vi "Parse Project Based Analysis.vi"(8 "error in (no error)":errorcluster, 11 "Element in":refnum<k20>) -> (0 "error out":errorcluster, 2 "Project Based Analysis":T1, 3 "Element out":refnum<k20>)   [LabVIEW 2020]
uses:
  <vilib>/xml/Close Reference(Node).vi
  <vilib>/xml/NI_XML.lvlib
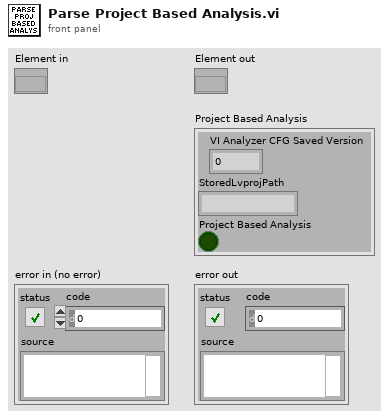
[diagram p1: front panel]
types:
  T1 = cluster{"VI Analyzer CFG Saved Version":u16, "StoredLvprojPath":string, "Project Based Analysis":bool}
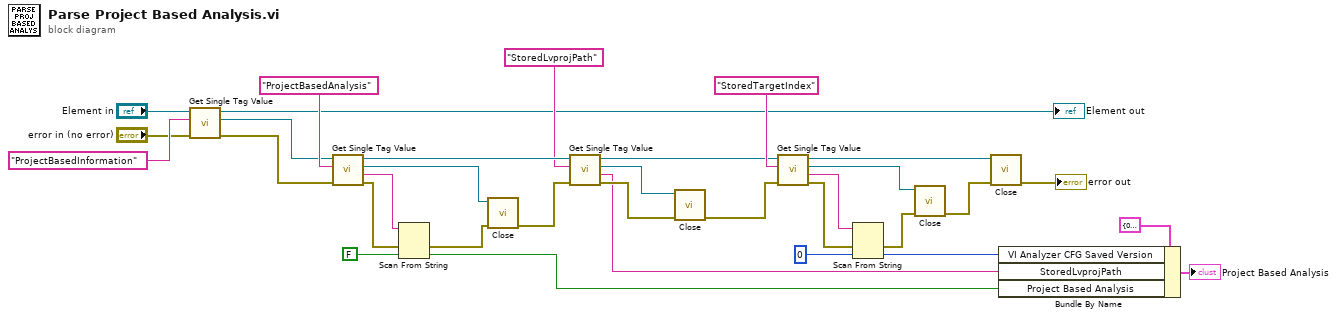
[diagram p0: block diagram]
diagram:
  n1 = call <vilib>:"Get Single Tag Value.vi"("Error In"="error in (no error)", "Tag Name"="ProjectBasedInformation", "Element In"="Element in") -> ("Error Out"=w2:errorcluster, "Tag Reference"=w5:refnum<k20>, "Element Out"=→"Element out":refnum<k20>)  [unwired: 5 in, 1 out]
  n2 = call <vilib>:"Get Single Tag Value.vi"("Error In"=w2, "Tag Name"="ProjectBasedAnalysis", "Element In"=w5) -> ("Error Out"=w18:errorcluster, "Tag Value"=w23:string, "Tag Reference"=w33:refnum<k20>, "Element Out"=w15:refnum<k20>)  [unwired: 5 in]
  n3 = Scan From String(input string=w23, error in=w18, default 1=FALSE) -> (error out=w31:errorcluster, output 1=w9:bool)  [unwired: 2 in, 2 out]
  n4 = call-poly <vilib>:"Close.vi"("error in (no error)"=w31, "node"=w33) -> ("error out"=w32:errorcluster)  [unwired: 7 in]
  n5 = call <vilib>:"Get Single Tag Value.vi"("Error In"=w32, "Tag Name"="StoredLvprojPath", "Element In"=w15) -> ("Error Out"=w26:errorcluster, "Tag Value"=w10:string, "Tag Reference"=w25:refnum<k20>, "Element Out"=w16:refnum<k20>)  [unwired: 5 in]
  n6 = call-poly <vilib>:"Close.vi"("error in (no error)"=w26, "node"=w25) -> ("error out"=w30:errorcluster)  [unwired: 7 in]
  n7 = call <vilib>:"Get Single Tag Value.vi"("Error In"=w30, "Tag Name"="StoredTargetIndex", "Element In"=w16) -> ("Error Out"=w20:errorcluster, "Tag Value"=w24:string, "Tag Reference"=w29:refnum<k20>, "Element Out"=w22:refnum<k20>)  [unwired: 5 in]
  n8 = Scan From String(input string=w24, error in=w20, default 1=u16 0 ("VI Analyzer CFG Saved Version")) -> (error out=w27:errorcluster, output 1=w11:u16)  [unwired: 2 in, 2 out]
  n9 = call-poly <vilib>:"Close.vi"("error in (no error)"=w27, "node"=w29) -> ("error out"=w28:errorcluster)  [unwired: 7 in]
  n10 = call-poly <vilib>:"Close.vi"("error in (no error)"=w28, "node"=w22) -> ("error out"=→"error out":errorcluster)  [unwired: 7 in]
  n11 = Bundle By Name(cluster=T1 {"VI Analyzer CFG Saved Version"=0, "StoredLvprojPath"="", "Project Based Analysis"=FALSE} ("output cluster"), "VI Analyzer CFG Saved Version"=w11, "StoredLvprojPath"=w10, "Project Based Analysis"=w9) -> (→"Project Based Analysis":T1)
